vi "generate_DAC_voltages_simple.vi"(7 "focus mode?":bool, 8 "derived values":T1, 9 "scan specification":T4={"x amplitude"=0, "x resolution (pixels)"=0, "x offset fly-forward (iterations)"=0, "x offset fly-back (iterations)"=0, "y resolution (nr. of lines)"=0, "y step size"=0, "iterations per pixel"=0, "number of frames"=0, "y offset (pixels)"=0, "number of y-brake lines  (before y-fly-back)"=0, "number y-brake lines (after y-fly-back)"=0, "number of y-fly-back steps"=8, "lines per z step"=0, "number of z/intensity tuples"=0, "number of repetitions (volumes or planes)"=0, "z step size derived"=0, "choose the beginning of z scan"=FALSE, "number of frames (settings)"=0, "FPGA trajectory?"=FALSE}, 10 "counter cluster in":T2, 11 "resonant trigger":bool) -> (0 "acquire?":bool, 1 "fly-back acquisition phase?":bool, 2 "counter cluster out":T2, 3 "DAC voltages":T3 {"ch6" max=4095 step=1; "ch5" max=4095 step=1; "ch4" max=4095 step=1; "ch3" max=4095 step=1; "ch2" max=4095 step=1; "ch1" max=4095 step=1; "ch0" max=4095 step=1})   [LabVIEW 2010]
uses:
  scan_specification_cluster.ctl
  common_typedefs/DAC_voltage_cluster.ctl
  counter_cluster.ctl
  derived_values_cluster.ctl
panel:
  out "coerced(x) 2":u16
  out "unsigned 16bit integer":u16
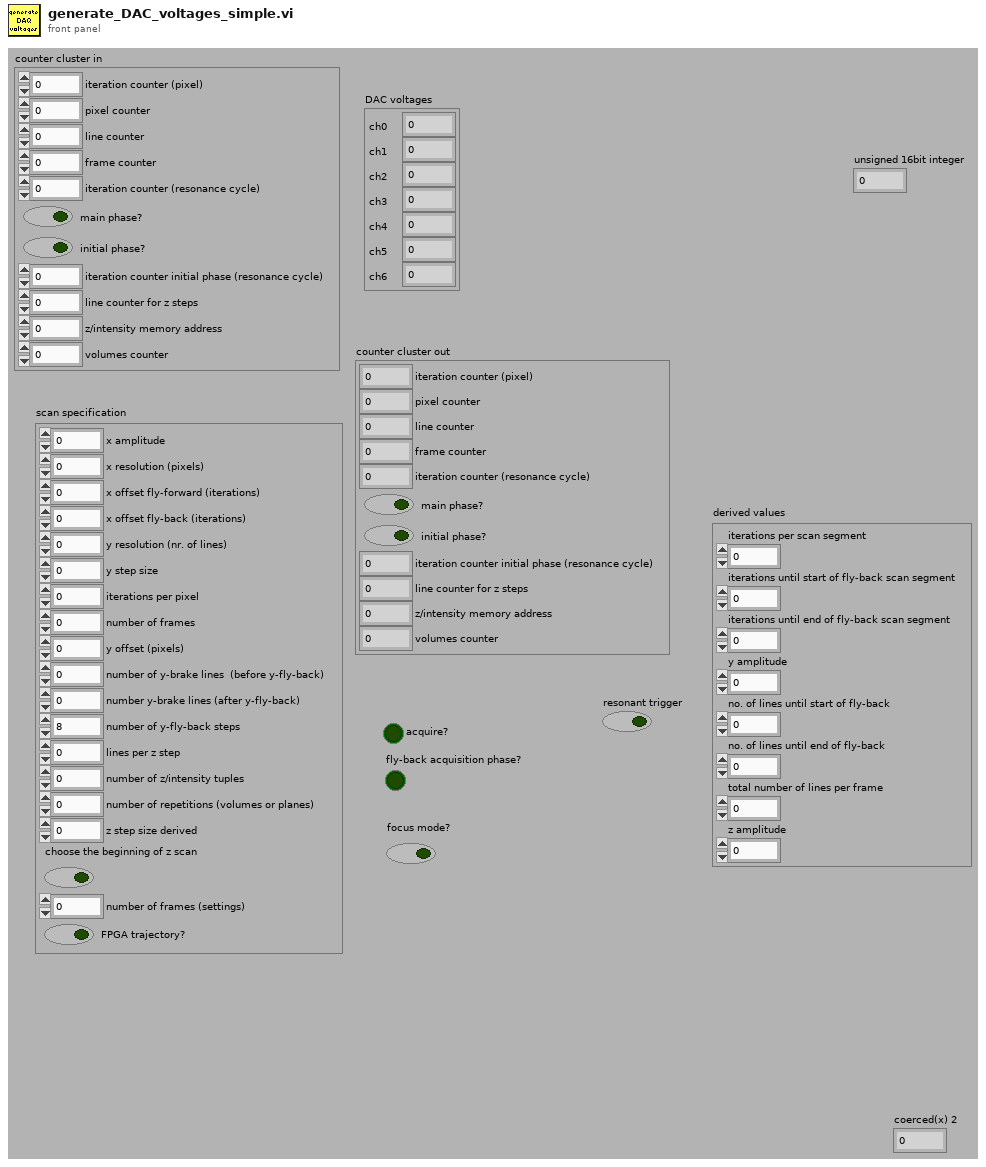
[diagram p1: front panel]
types:
  T1 = typedef "derived_values_cluster.ctl" = cluster{"iterations per scan segment":u16, "iterations until start of fly-back scan segment":u16, "iterations until end of fly-back scan segment":u16, "y amplitude":u16, "no. of lines until start of fly-back":u16, "no. of lines until end of fly-back":u16, "total number of lines per frame ":u16, "z amplitude":u16}
  T2 = typedef "counter_cluster.ctl" = cluster{"iteration counter (pixel)":u16, "pixel counter":u16, "line counter":u16, "frame counter":u16, "iteration counter (resonance cycle)":u16, "main phase?":bool, "initial phase?":bool, "iteration counter initial phase (resonance cycle)":u16, "line counter for z steps":u16, "z/intensity memory address":u32, "volumes counter":u16}
  T3 = typedef "DAC_voltage_cluster.ctl" = cluster{"ch0":u16, "ch1":i16, "ch2":i16, "ch3":u16, "ch4":u16, "ch5":u16, "ch6":u16}
  T4 = typedef "scan_specification_cluster.ctl" = cluster{"x amplitude":u16, "x resolution (pixels)":u16, "x offset fly-forward (iterations)":u16, "x offset fly-back (iterations)":u16, "y resolution (nr. of lines)":u16, "y step size":u16, "iterations per pixel":u16, "number of frames":i32, "y offset (pixels)":u16, "number of y-brake lines  (before y-fly-back)":u16, "number y-brake lines (after y-fly-back)":u16, "number of y-fly-back steps":u16, "lines per z step":u16, "number of z/intensity tuples":u16, "number of repetitions (volumes or planes)":i32, "z step size derived":u16, "choose the beginning of z scan":bool, "number of frames (settings)":i32, "FPGA trajectory?":bool}
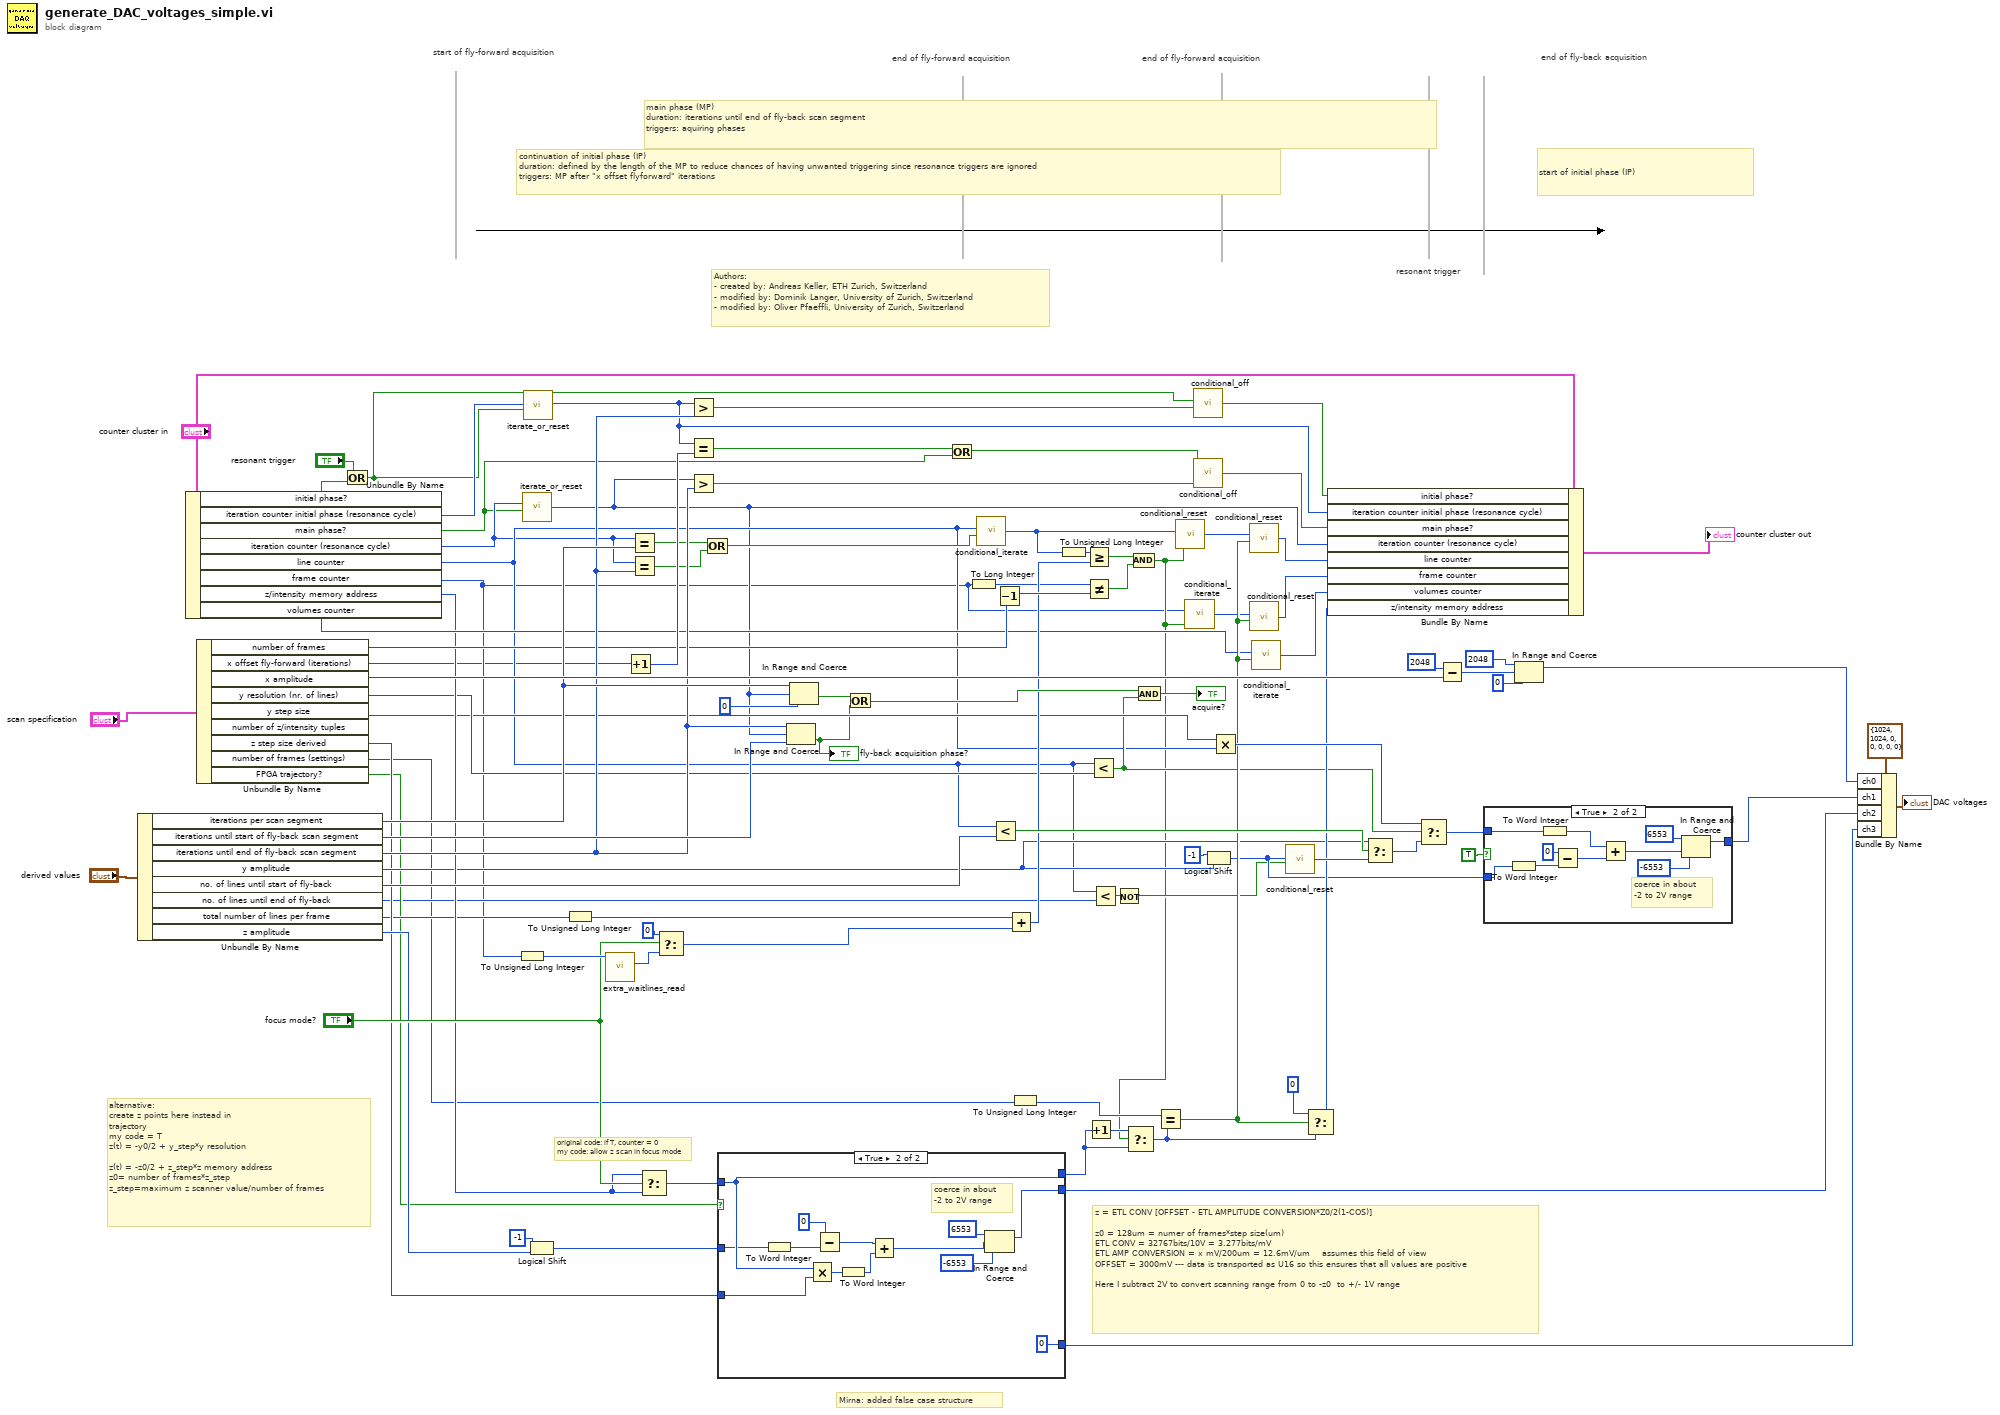
[diagram p0: block diagram]
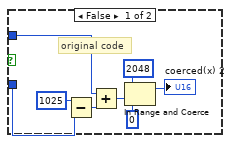
[diagram p2: hidden frame]
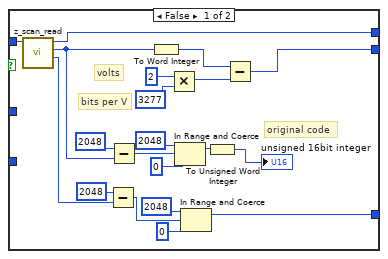
[diagram p3: hidden frame]
diagram:
  # "z = ETL CONV [OFFSET - ETL AMPLITUDE CONVERSION*Z0/2(1-COS)]\n\nz0 = 128um = numer of frames*step size(um)\nETL CONV = 32767bits/10V = 3.277bits/mV\nETL AMP CONVERSION = x mV/200um = 12.6mV/um    assumes this field of view\nOFFSET = 3000mV --- data is transported as U16 so this ensures that all values are positive\n\nHere I subtract 2V to convert scanning range from 0 to -z0  to +/- 1V range"
  # "alternative:\ncreate z points here instead in \ntrajectory\nmy code = T\nz(t) = -y0/2 + y_step*y resolution\n\nz(t) = -z0/2 + z_step*z memory address\nz0= number of frames*z_step\nz_step=maximum z scanner value/number of frames"
  # "original code: if T, counter = 0\nmy code: allow z scan in focus mode"
  # "Mirna: added false case structure"
  # "start of initial phase (IP)"
  # "continuation of initial phase (IP)\nduration: defined by the length of the MP to reduce chances of having unwanted triggering since resonance triggers are ignored\ntriggers: MP after \"x offset flyforward\" iterations"
  # "end of fly-back acquisition"
  # "end of fly-forward acquisition"
  # "end of fly-forward acquisition"
  # "start of fly-forward acquisition"
  # "main phase (MP)\nduration: iterations until end of fly-back scan segment\ntriggers: aquiring phases"
  # "resonant trigger"
  # "Authors: \n- created by: Andreas Keller, ETH Zurich, Switzerland\n- modified by: Dominik Langer, University of Zurich, Switzerland\n- modified by: Oliver Pfaeffli, University of Zurich, Switzerland"
  n1 = Unbundle By Name("derived values") -> ("iterations per scan segment"=w75:u16, "iterations until start of fly-back scan segment"=w78:u16, "iterations until end of fly-back scan segment"=w63:u16, "y amplitude"=w28:u16, "no. of lines until start of fly-back"=w66:u16, "no. of lines until end of fly-back"=w13:u16, "total number of lines per frame"=w24:u16, "z amplitude"=w26:u16)
  n2 = Unbundle By Name("counter cluster in") -> ("initial phase?"=w77:bool, "iteration counter initial phase (resonance cycle)"=w73:u16, "main phase?"=w8:bool, "iteration counter (resonance cycle)"=w10:u16, "line counter"=w11:u16, "frame counter"=w3:u16, "z/intensity memory address"=w32:u32, "volumes counter"=w41:u16)
  n3 = Unbundle By Name("scan specification") -> ("number of frames"=w48:i32, "x offset fly-forward (iterations)"=w1:u16, "x amplitude"=w82:u16, "y resolution (nr. of lines)"=w31:u16, "y step size"=w27:u16, "z step size derived"=w25:u16, "number of frames (settings)"=w4:i32, "FPGA trajectory?"=w15:bool)  [unwired: 1 out]
  n4 = Or(x="resonant trigger", y=w77) -> (x .or. y?=w71:bool)
  n5 = To Unsigned Long Integer(number=w3) -> (unsigned 32bit integer=w54:u32)
  n6 = call "iterate_or_reset.vi"("iterate?"=w8, "number in"=w10) -> ("number out"=w7:u16)  [unwired: 4 in]
  n7 = call "iterate_or_reset.vi"("iterate?"=w71, "number in"=w73) -> ("number out"=w23:u16)  [unwired: 4 in]
  n8 = Logical Shift(y=i16 -1 ("n"), x=w26) -> (x << y=w38:u16)
  n9 = To Unsigned Long Integer(number=w24) -> (unsigned 32bit integer=w2:u32)
  n10 = call "extra_waitlines_read.vi"("address extra waitlines IN"=w54) -> ("extra waitline data"=w44:u32)  [unwired: 9 in, 1 out]
  n11 = Increment(x=w1) -> (x+1=w65:u16)
  n12 = Equal?(x=w10, y=w75) -> (x = y?=w61:bool)
  n13 = Equal?(x=w10, y=w63) -> (x = y?=w62:bool)
  n14 = Select(t=w32, s="focus mode?", f=w32) -> (s? t:f=w33:u32)
  n15 = Select(t=u32 0, s="focus mode?", f=w44) -> (s? t:f=w43:u32)
  n16 = Greater?(x=w23, y=w63) -> (0:w64:bool)
  n17 = Equal?(x=w23, y=w65) -> (x = y?=w72:bool)
  n18 = Greater?(x=w7, y=w63) -> (0:w69:bool)
  n19 = Or(x=w61, y=w62) -> (x .or. y?=w56:bool)
  n20 = case shown="True" w15 {
    tunnel: [w110 u16 0 ("intensity")] -> w35
    tunnel: [w117 w127] -> w55
    tunnel: [w101 w118] -> w34
    tunnel: w33 -> [w116 w127]
    tunnel: w38 -> [_ w119]
    tunnel: w25 -> [_ w128]
    frame False {
      # "bits per V"
      # "volts"
      # "original code"
      n21 = call "z_scan_read.vi"("address in"=w116) -> ("intensity"=w113:u16, "z-value"=w103:i16, "address out"=w117:u32)  [unwired: 8 in]
      n22 = Subtract(x=i16 2048, y=w113) -> (x-y=w109:u16)
      n23 = Subtract(x=i16 2048, y=w103) -> (x-y=w105:i16)
      n24 = To Word Integer(number=w103) -> (16bit integer=w102:i16)
      n25 = Multiply(x=i16 2 ("y"), y=i16 3277) -> (x*y=w99:i16)
      n26 = In Range and Coerce(upper limit=i16 2048, x=w105, lower limit=i16 0) -> (coerced(x)=w106:i16)  [unwired: 1 out]
      n27 = In Range and Coerce(upper limit=u16 2048, x=w109, lower limit=u16 0) -> (coerced(x)=w110:u16)  [unwired: 1 out]
      n28 = To Unsigned Word Integer(number=w106) -> (unsigned 16bit integer=→"unsigned 16bit integer":u16)
      n29 = Subtract(x=w102, y=w99) -> (x-y=w101:i16)
    }
    frame True {
      # "coerce in about\n-2 to 2V range"
      n30 = To Word Integer(number=w119) -> (16bit integer=w124:i16)
      n31 = Multiply(x=w127, y=w128) -> (x*y=w125:u32)
      n32 = Subtract(x=i16 0, y=w124) -> (x-y=w126:i16)
      n33 = To Word Integer(number=w125) -> (16bit integer=w123:i16)
      n34 = Add(x=w126, y=w123) -> (x+y=w120:i16)
      n35 = In Range and Coerce(upper limit=i16 6553, x=w120, lower limit=i16 -6553) -> (coerced(x)=w118:i16)  [unwired: 1 out]
    }
  }
  n36 = In Range and Coerce(upper limit=w63, x=w7, lower limit=w78) -> (In Range?=w16:bool)  [unwired: 1 out]
  "fly-back acquisition phase?" <- w16
  n37 = In Range and Coerce(upper limit=w75, x=w7, lower limit=u16 0) -> (In Range?=w90:bool)  [unwired: 1 out]
  n38 = Or(x=w90, y=w16) -> (x .or. y?=w81:bool)
  n39 = Or(x=w72, y=w8) -> (x .or. y?=w37:bool)
  n40 = To Long Integer(number=w3) -> (32bit integer=w6:i32)
  n41 = call "conditional_iterate.vi"("iterate?"=w56, "number in"=w11) -> ("number out"=w9:u16)  [unwired: 4 in]
  n42 = Less?(x=w11, y=w66) -> (x < y?=w96:bool)
  n43 = Decrement(x=w48) -> (x-1=w47:i32)
  n44 = Add(x=w2, y=w43) -> (x+y=w45:u32)
  n45 = To Unsigned Long Integer(number=w4) -> (unsigned 32bit integer=w59:u32)
  n46 = To Unsigned Long Integer(number=w9) -> (unsigned 32bit integer=w14:u32)
  n47 = Greater Or Equal?(x=w14, y=w45) -> (x >= y?=w49:bool)
  n48 = Not Equal?(x=w6, y=w47) -> (x != y?=w12:bool)
  n49 = Increment(x=w55) -> (x+1=w60:u32)
  n50 = Less?(x=w11, y=w31) -> (x < y?=w19:bool)
  n51 = Less?(x=w11, y=w13) -> (x < y?=w80:bool)
  n52 = Not(x=w80) -> (.not. x?=w17:bool)
  n53 = And(x=w49, y=w12) -> (x .and. y?=w5:bool)
  n54 = Select(t=w60, s=w5, f=w55) -> (s? t:f=w58:u32)
  n55 = And(x=w81, y=w19) -> (x .and. y?=→"acquire?":bool)
  n56 = Equal?(x=w59, y=w58) -> (x = y?=w46:bool)
  n57 = call "conditional_reset.vi"("reset?"=w5, "number in"=w9) -> ("number out"=w51:u16)  [unwired: 4 in]
  n58 = call "conditional_iterate.vi"("iterate?"=w5, "number in"=w3) -> ("number out"=w29:u16)  [unwired: 4 in]
  n59 = call "conditional_off.vi"("switch off?"=w64, "boolean in"=w71) -> ("boolean out"=w70:bool)  [unwired: 4 in]
  n60 = call "conditional_off.vi"("switch off?"=w69, "boolean in"=w37) -> ("boolean out"=w68:bool)  [unwired: 4 in]
  n61 = Logical Shift(y=i16 -1 ("n"), x=w28) -> (x << y=w18:u16)
  n62 = Multiply(x=w27, y=w11) -> (x*y=w95:u16)
  n63 = call "conditional_reset.vi"("reset?"=w46, "number in"=w51) -> ("number out"=w50:u16)  [unwired: 4 in]
  n64 = call "conditional_reset.vi"("reset?"=w46, "number in"=w29) -> ("number out"=w30:u16)  [unwired: 4 in]
  n65 = call "conditional_iterate.vi"("iterate?"=w46, "number in"=w41) -> ("number out"=w52:u16)  [unwired: 4 in]
  n66 = call "conditional_reset.vi"("reset?"=w17, "number in"=w18) -> ("number out"=w67:u16)  [unwired: 4 in]
  n67 = Select(t=u32 0, s=w46, f=w58) -> (s? t:f=w53:u32)
  n68 = Bundle By Name(cluster="counter cluster in", "initial phase?"=w70, "iteration counter initial phase (resonance cycle)"=w23, "main phase?"=w68, "iteration counter (resonance cycle)"=w7, "line counter"=w50, "frame counter"=w30, "volumes counter"=w52, "z/intensity memory address"=w53) -> (→"counter cluster out":T2)
  n69 = Select(t=w28, s=w96, f=w67) -> (s? t:f=w20:u16)
  n70 = Select(t=w95, s=w19, f=w20) -> (s? t:f=w22:u16)
  n71 = Subtract(x=u16 2048, y=w82) -> (x-y=w86:u16)
  n72 = case shown="True" TRUE {
    tunnel: [_ w141] -> w36
    tunnel: w18 -> [w131 w140]
    tunnel: w22 -> [w132 w139]
    frame False {
      # "original code"
      n73 = Subtract(x=u16 1025, y=w131) -> (x-y=w134:u16)
      n74 = Add(x=w132, y=w134) -> (x+y=w133:u16)
      n75 = In Range and Coerce(upper limit=u16 2048, x=w133, lower limit=u16 0) -> (coerced(x)=→"coerced(x) 2":u16)  [unwired: 1 out]
    }
    frame True {
      # "coerce in about\n-2 to 2V range"
      n76 = To Word Integer(number=w140) -> (16bit integer=w146:i16)
      n77 = To Word Integer(number=w139) -> (16bit integer=w145:i16)
      n78 = Subtract(x=i16 0, y=w146) -> (x-y=w147:i16)
      n79 = Add(x=w145, y=w147) -> (x+y=w142:i16)
      n80 = In Range and Coerce(upper limit=i16 6553, x=w142, lower limit=i16 -6553) -> (coerced(x)=w141:i16)  [unwired: 1 out]
    }
  }
  n81 = In Range and Coerce(upper limit=u16 2048, x=w86, lower limit=u16 0) -> (coerced(x)=w85:u16)  [unwired: 1 out]
  n82 = Bundle By Name(cluster=T3 {"ch0"=1024, "ch1"=1024, "ch2"=0, "ch3"=0, "ch4"=0, "ch5"=0, "ch6"=0} ("DAC voltage"), "ch0"=w85, "ch1"=w36, "ch2"=w34, "ch3"=w35) -> (→"DAC voltages":T3)
